vi "check_frequency_sweepI_parameters.vi"(8 "error in (no error)":errorcluster, 10 "Frequency Sweep I Parameters":T1={"f_start (Hz)"=0.0, "f_end (Hz)"=0.0, "Number of steps"=2, "Total time (s)"=0.0, "fc (Hz)"=2000.0, "Modulation Depth (0.0 %)"=0.0, "Channel (1:Channel 1)"=2, "amp (V)"=1.0, "DC Offset (V)"=0.0} {"DC Offset (V)" min=-20.0 max=20.0 format="%#_13g"; "amp (V)" min=0.0 max=20.0 format="%#_13g"; "Channel (1:Channel 1)" items=["Channel 1"=1, "Channel 2"=2]; "Modulation Depth (0.0 %)" min=0.0 max=120.0 format="%.1f"; "fc (Hz)" min=0.0 format="%#_13g"; "Total time (s)" min=0.0; "Number of steps" min=2; "f_end (Hz)" min=0.0; "f_start (Hz)" min=0.0}) -> (0 "error out":errorcluster, 1 "Array":dbl[](array[numeric]), 2 "Entered Values OK":bool)   [LabVIEW 2024, in "Sweep.lvlib"]
uses:
  Sweep.lvlib
  Type Definitions/Frequency_sweep_I Parameters.ctl
panel:
  out "fc (Hz)":dbl
  out "Number of frequencies":i32
  out "Total time T (s)":dbl
  out "Channel (1:Channel 1)":i32
  out "Modulation Depth (0.0 %)":dbl
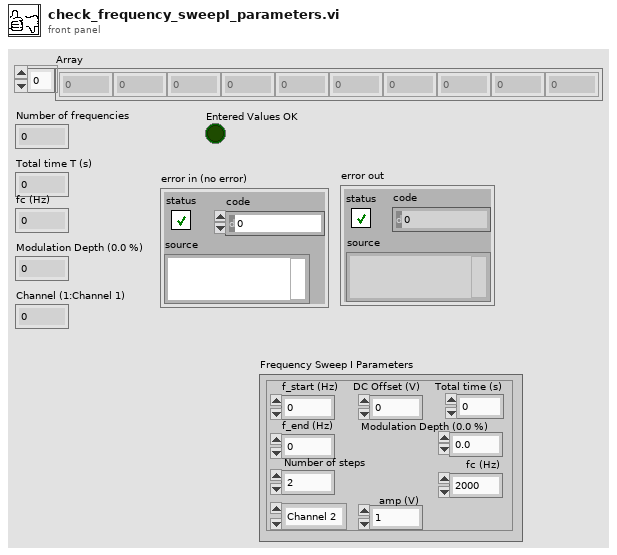
[diagram p1: front panel]
types:
  T1 = typedef "Frequency_sweep_I Parameters.ctl" = cluster{"f_start (Hz)":dbl, "f_end (Hz)":dbl, "Number of steps":i32, "Total time (s)":dbl, "fc (Hz)":dbl, "Modulation Depth (0.0 %)":dbl, "Channel (1:Channel 1)":i32, "amp (V)":dbl, "DC Offset (V)":dbl}
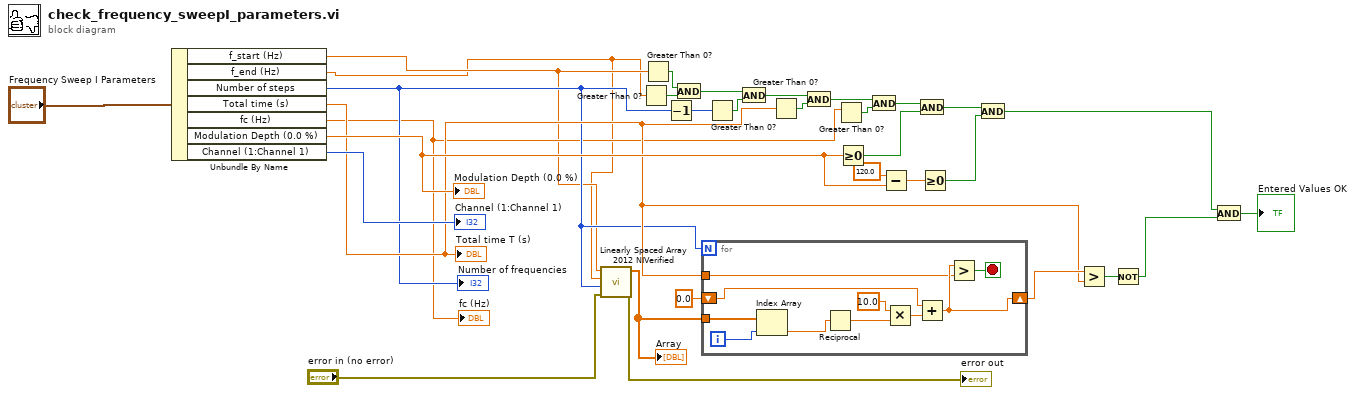
[diagram p0: block diagram]
diagram:
  n1 = Unbundle By Name("Frequency Sweep I Parameters") -> ("f_start (Hz)"=w2:dbl, "f_end (Hz)"=w1:dbl, "Number of steps"=w4:i32, "Total time (s)"=w5:dbl, "fc (Hz)"=w3:dbl, "Modulation Depth (0.0 %)"=w7:dbl, "Channel (1:Channel 1)"=→"Channel (1:Channel 1)":i32)
  "Modulation Depth (0.0 %)" <- w7
  "Total time T (s)" <- w5
  "Number of frequencies" <- w4
  "fc (Hz)" <- w3
  n2 = call "Linearly Spaced Array 2012 NIVerified.vi"("error in (no error)"="error in (no error)", "Number of Samples"=w4, "End"=w1, "Start"=w2) -> ("error out"=→"error out":errorcluster, "Array"=w28:dbl[])  [unwired: 6 in]
  "Array" <- w28
  n3 = Greater Than 0?(x=w1) -> (x > 0?=w20:bool)
  n4 = Greater Than 0?(x=w2) -> (x > 0?=w19:bool)
  n5 = Decrement(x=w4) -> (x-1=w15:i32)
  n6 = And(x=w19, y=w20) -> (x .and. y?=w21:bool)
  n7 = for {
    N: w4 -> [_]
    tunnel: w28 -> [w42]
    shift-right: [w36] -> w30
    shift-left: 0.0 -> [w37]
    tunnel: w5 -> [w33]
    i -> [w34]
    stop <- w35 stop-if-true
    n8 = Index Array "Index Array"(array=w42, index=w34) -> (element=w41:dbl)
    n9 = Reciprocal(x=w41) -> (1/x=w40:dbl)
    n10 = Multiply(x=10.0, y=w40) -> (x*y=w38:dbl)
    n11 = Add(x=w37, y=w38) -> (x+y=w36:dbl)
    n12 = Greater?(x=w36, y=w33) -> (0:w35:bool)
  }
  n13 = Greater Than 0?(x=w15) -> (x > 0?=w22:bool)
  n14 = And(x=w21, y=w22) -> (x .and. y?=w23:bool)
  n15 = Greater Than 0?(x=w5) -> (x > 0?=w24:bool)
  n16 = And(x=w23, y=w24) -> (x .and. y?=w25:bool)
  n17 = Greater Than 0?(x=w3) -> (x > 0?=w26:bool)
  n18 = Greater Or Equal To 0?(x=w7) -> (x >= 0?=w14:bool)
  n19 = And(x=w25, y=w26) -> (x .and. y?=w29:bool)
  n20 = Subtract(x=120.0, y=w7) -> (x-y=w11:dbl)
  n21 = And(x=w29, y=w14) -> (x .and. y?=w12:bool)
  n22 = Greater Or Equal To 0?(x=w11) -> (x >= 0?=w10:bool)
  n23 = And(x=w12, y=w10) -> (x .and. y?=w13:bool)
  n24 = Greater?(x=w30, y=w5) -> (0:w31:bool)
  n25 = Not(x=w31) -> (.not. x?=w32:bool)
  n26 = And(x=w13, y=w32) -> (x .and. y?=→"Entered Values OK":bool)
